vi "SPD Single Point Test Launcher.vi"() -> ()   [LabVIEW 2018]
uses:
  SPD Stand/typedefs/SPD.Stand state.ctl
  SPD Stand/typedefs/SPD.Stand Tabs.ctl
  Instruments/SPD HID Interface/hidSPDLibForLabView/LibVIs/hidSPD Controls/hidSPD SPD Type.ctl
  Instruments/SPD HID Interface/hidSPDLibForLabView/hidSPDLibForLabView.lvlib
  SPD Stand/typedefs/SPD.Queues.ctl
  SPD Stand/typedefs/SPD.Meas Grid.ctl
  <vilib>/Utility/config.llb/Config Data RefNum.ctl
  <vilib>/Utility/config.llb/NI_LVConfig.lvlib
  SPD Stand/ConfigFile/SPD.Config File ctrl.ctl
  SPD Stand/typedefs/SPD.Events.ctl
  Instruments/LeCroy SDA830/typedefs/LeCroy.Session.ctl
  Instruments/KeySight 8164B/KeySight 8164B LAN InstrLib/typedefs/KeySight 8164B control.ctl
  Instruments/KeySight 8164B/KeySight 8164B LAN InstrLib.lvlib
  Instruments/KeySight 53230A/typedefs/FreqC.Session.ctl
  Instruments/KC705 DevBoard/typedefs/DevB.Session.ctl
  Instruments/SPD HID Interface/hidSPDLibForLabView/LibVIs/hidSPD Controls/hidSPD Controller.ctl
  Instruments/SPD HID Interface/hidSPDLibForLabView/LibVIs/hidSPD Controls/hidSPD Device Session.ctl
  SPD Stand/typedefs/SPD.Stand Ctrl.ctl
  Instruments/SPD HID Interface/hidSPDLibForLabView/LibVIs/hidSPD Controls/hidSPD.STB Frequency.ctl
  Instruments/SPD HID Interface/hidSPDLibForLabView/LibVIs/hidSPD Controls/hidSPD SPD Diod Case.ctl
  Instruments/SPD HID Interface/hidSPDLibForLabView/LibVIs/hidSPD Controls/hidSPD.SPD specification.ctl
panel:
  out "Console":string caption="Консоль"
  out "test tabs":T1
  in  "HW.Ignore Equipment Tests":bool
  out "HW.KC Selftest":bool caption="Пройдено"
  in  "HW.KC705 Test":bool
  out "HW.PowerSource Selftest":bool caption="Пройдено"
  in  "HW.PowerSource Test":bool
  out "HW.Laser Selftest":bool caption="Пройдено"
  in  "HW.Laser Test":bool
  out "HW.Scope Selftest":bool caption="Пройдено"
  in  "HW.Scope Test":bool
  out "HW.8164B Selftest":bool caption="Пройдено"
  in  "HW.8164B Test":bool
  out "HW.FreqC Selftest":bool caption="Пройдено"
  in  "HW.FreqC Test":bool
  in  "Equipment.Connect":bool
  out "DevBSession.connected":bool caption="КС705"
  out "8164BSession.connected":bool caption="8164B"
  out "FreqCSession.connected":bool caption="Частотомер"
  out "LeCroySession.connected":bool caption="Осциллограф"
  in  "SPD.Type":T2=enum."Free Run" caption="Тип детектора"
  out "Diod T":sgl(graph) caption="Температура Диода"
  out "Heatsinck T":sgl(graph) caption="Температура Радиатора"
  in  "SPD.connect":bool
  out "hidSPDSession.connected":bool caption="Детектор подключен"
  out "spdDeviceSession.spdName":string caption="Имя Детектора"
  out "SPD.ready":bool caption="Вышел на режим"
  in  "TSet":sgl=-45.0 format="%#_g, Град С"
  in  "HV_bias":sgl=40.0 format="%#_g, В"
  in  "SPD.write":bool caption="Записать"
  out "PhaseTestProgress":dbl(slide) scale=0.0..1.0
  out "PhaseSetupGraph":cluster{dbl[], dbl[]}(graph) caption="Настройка Фазы Строба"
  out "HV_biasSetupGraph":cluster{dbl[], dbl[]}(graph) caption="Настройка Напряжения Смещения"
  out "Test.01_NoPulses Pass":bool caption="Отсутствие импульсов"
  in  "SPD.Tests":bool
  out "HV_BiasTestProgress":dbl(slide) scale=0.0..1.0
  out "Current Meas Progress":dbl(slide) caption="Измерение QE и TR" scale=0.0..1.0
  in  "Meas":bool
  out "Overall Meas Progress":dbl(slide) caption="Температура 1 из 1" scale=0.0..1.0
  out "Meas Time, min":dbl=nan format="%.2f"
  in  "SPMeas.Temprature":dbl=-45.0 caption="Температура"
  in  "SPMeas.Strobe_code":dbl=900.0 caption="Амплитуда Строба"
  in  "SPMeas.HV_bias":dbl=76.9 caption="Напряжение Смещения"
  out "Error Out":errorcluster
  out "SPD.Result":T3
  out "HW.Error Out":errorcluster
  in  "App.stop":bool
  in  "Back":bool
  in  "Next":bool
  # "Расширенные тесты оборудования"
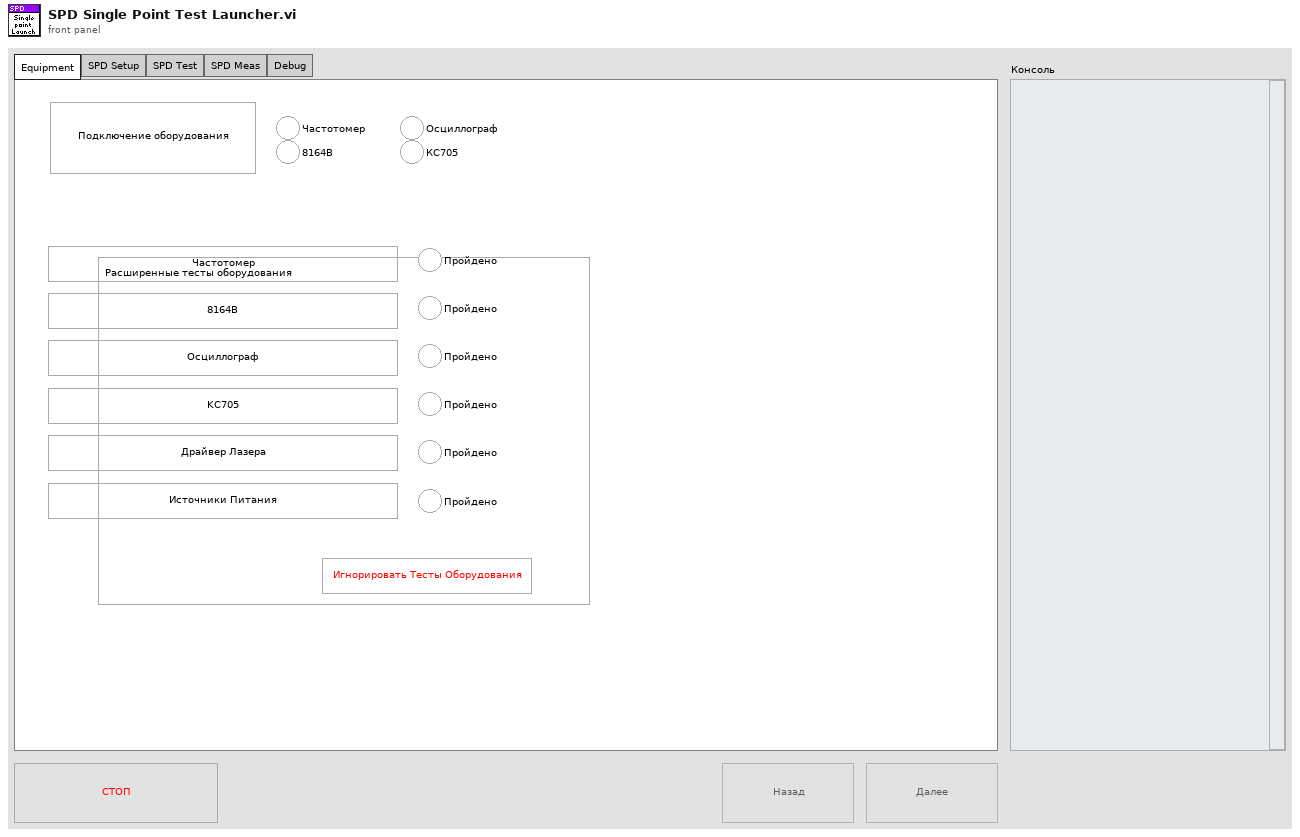
[diagram p1: front panel]
types:
  T1 = typedef "SPD.Stand Tabs.ctl" = enum32{"Equipment", "SPD Setup", "SPD Test", "SPD Meas", "Debug"}
  T2 = typedef "hidSPDLibForLabView.lvlib/hidSPD SPD Type.ctl" = enum16{"Unknown", "Free Run", "Gate"}
  T3 = typedef "SPD.Meas Grid.ctl" = cluster{"DateTime":string, "DT":dbl[], "Insensitivity":dbl[], "Temprature":dbl[], "Stb_code":dbl[], "HV_Bias":dbl[][][][]}
  T4 = typedef "SPD.Stand Ctrl.ctl" = cluster{"spdDeviceSession":T5, "DevBSession":T10, "FreqCSession":T11, "8164BSession":T12, "LeCroySession":T13, "Events":T14, "configFile":T15, "SPD.Meas Grid":T3, "SPD.Queues":T17, "Console":refnum<vi>}
  T5 = typedef "hidSPDLibForLabView.lvlib/hidSPD Device Session.ctl" = cluster{"spdRef":u64, "connected":bool, "spdName":string, "specification":T6, "hidSPD.Controller":T9, "hidSPD.Sturtup Values":T9}
  T6 = typedef "hidSPDLibForLabView.lvlib/hidSPD.SPD specification.ctl" = cluster{"diod case":T7, "type":T2, "frequency":T8}
  T7 = typedef "hidSPDLibForLabView.lvlib/hidSPD SPD Diod Case.ctl" = enum16{"Unknown", "default", "butterfly"}
  T8 = typedef "hidSPDLibForLabView.lvlib/hidSPD.STB Frequency.ctl" = enum16{"Unknown", "312", "1250"}
  T9 = typedef "hidSPDLibForLabView.lvlib/hidSPD Controller.ctl" = cluster{"TSet":sgl, "HV_bias":sgl, "DDS_stb_code":u16}
  T10 = typedef "DevB.Session.ctl" = cluster{"DevBRef":refnum<visa-resource-name>, "connected":bool}
  T11 = typedef "FreqC.Session.ctl" = cluster{"FreqCRef":refnum<visa-resource-name>, "timeout":dbl, "Gate":dbl, "connected":bool}
  T12 = typedef "KeySight 8164B LAN InstrLib.lvlib/KeySight 8164B control.ctl" = cluster{"Connection ID":refnum<k5>, "Connected":bool, "Info":string, "Slots Info":string[]}
  T13 = typedef "LeCroy.Session.ctl" = cluster{"LeCroySession":refnum<visa-resource-name>, "connected":bool}
  T14 = typedef "SPD.Events.ctl" = cluster{"DCRTest":refnum<user-event>, "Stop":refnum<user-event>}
  T15 = typedef "SPD.Config File ctrl.ctl" = cluster{"configFile ref":T16, "configFile path":path, "equipmentFile ref":T16}
  T16 = typedef "NI_LVConfig.lvlib/Config Data RefNum.ctl" = refnum<k1>
  T17 = typedef "SPD.Queues.ctl" = cluster{"state queue":refnum<queue>}
  T18 = enum8{"Enabled", "Disabled", "Disabled and Grayed Out"}
  T19 = typedef "SPD.Stand state.ctl" = enum16{"idle", "HW.Conect", "HW.FreqC selftest", "HW.8164B selftest", "HW.Scope selftest", "HW.KC705 selftest", "HW.Laser test", "HW.Power source test", "SPD.connect", "SPD.set type", "SPD.write", "SPD.read", "SPD.tests", "Btf.DT&Insens", "Meas.Grid update", "Meas", "App.Handle Error", "App.Stop"}
  T20 = typedef "hidSPDLibForLabView.lvlib/hidSPD SPD Type.ctl" = enum16{"Unknown", "Free Run", "Gate_312", "Gate_1250"}
  T21 = typedef "SPD.Meas Result.ctl" = cluster{"HV_Bias":dbl[][][], "Stb_code":dbl[], "Temprature":dbl[], "Data":dbl[][][][], "DateTime":string}
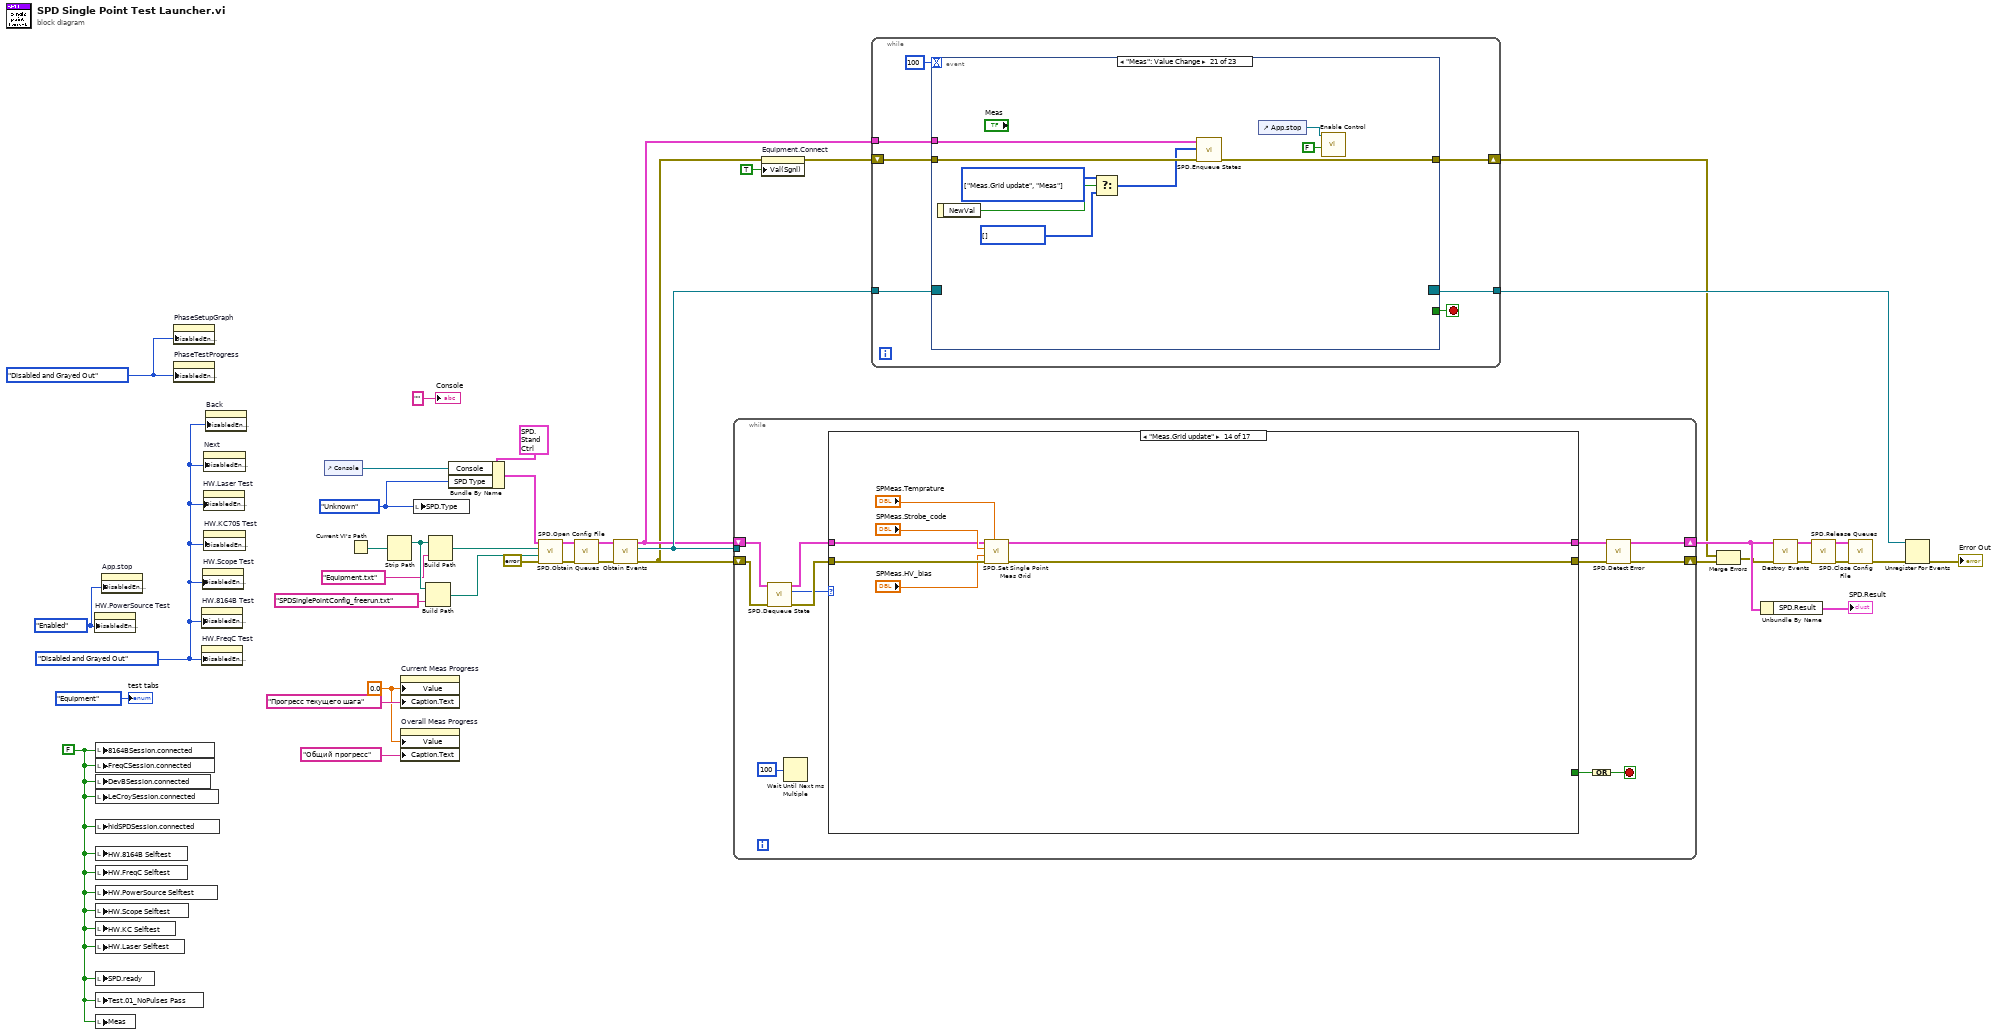
[diagram p0: block diagram]
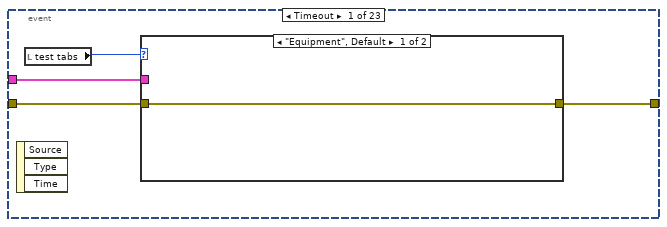
[diagram p2: hidden frame]
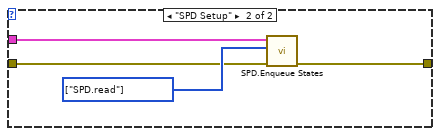
[diagram p3: hidden frame]
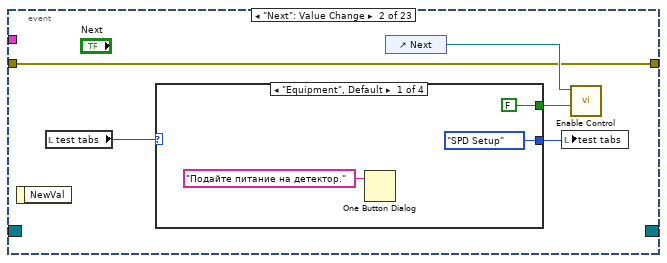
[diagram p4: hidden frame]
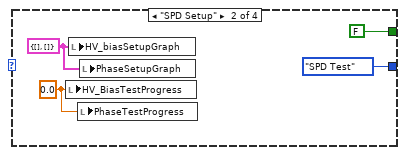
[diagram p5: hidden frame]
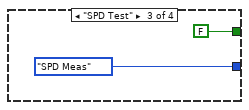
[diagram p6: hidden frame]
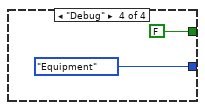
[diagram p7: hidden frame]
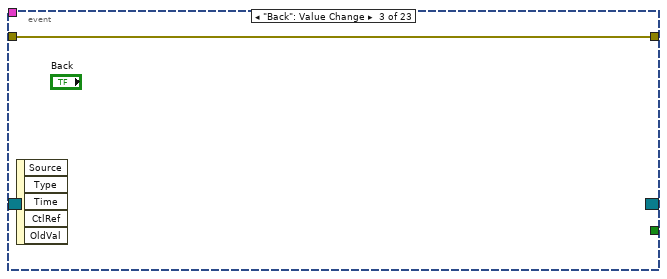
[diagram p8: hidden frame]
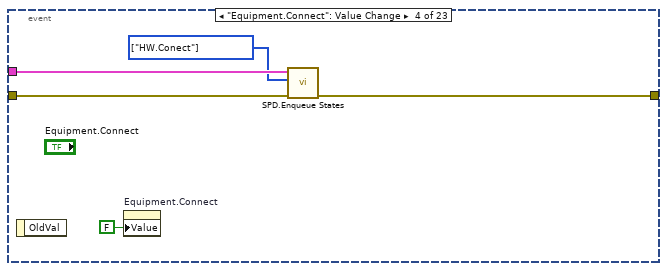
[diagram p9: hidden frame]
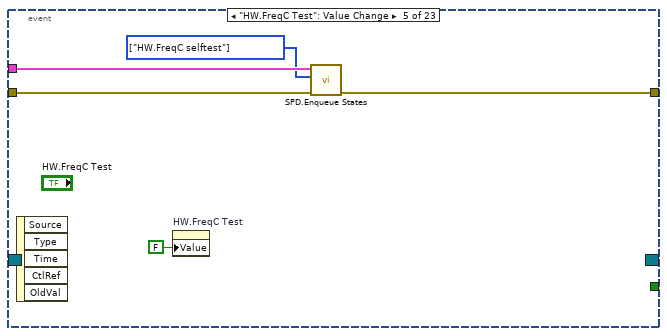
[diagram p10: hidden frame]
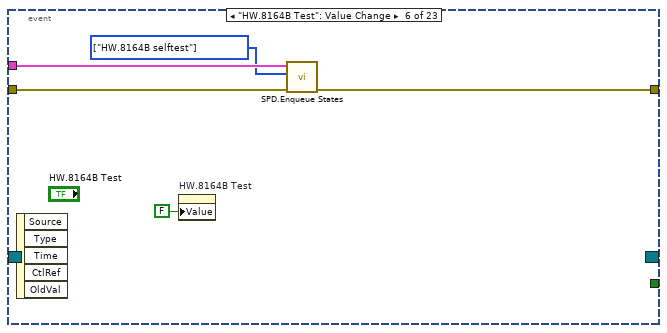
[diagram p11: hidden frame]
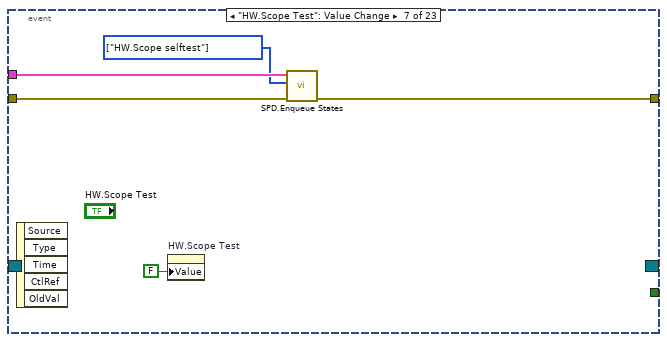
[diagram p12: hidden frame]
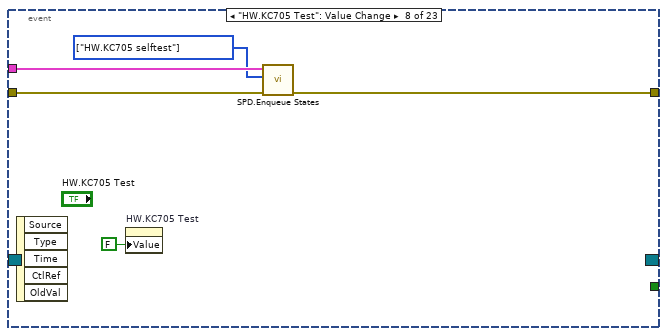
[diagram p13: hidden frame]
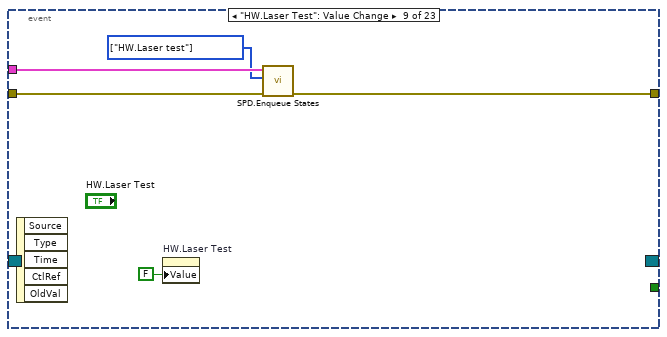
[diagram p14: hidden frame]
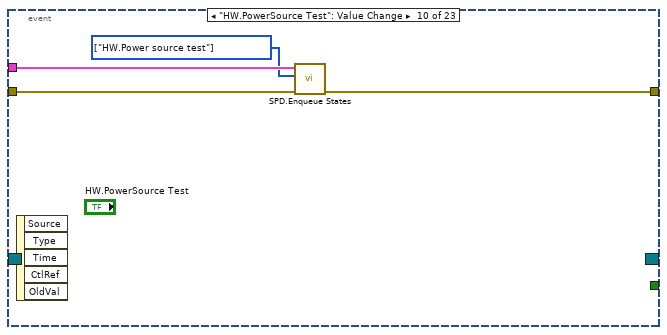
[diagram p15: hidden frame]
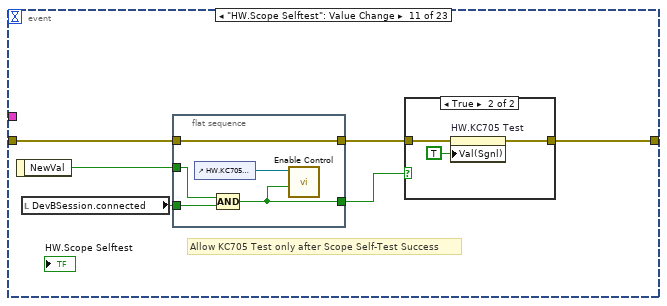
[diagram p16: hidden frame]
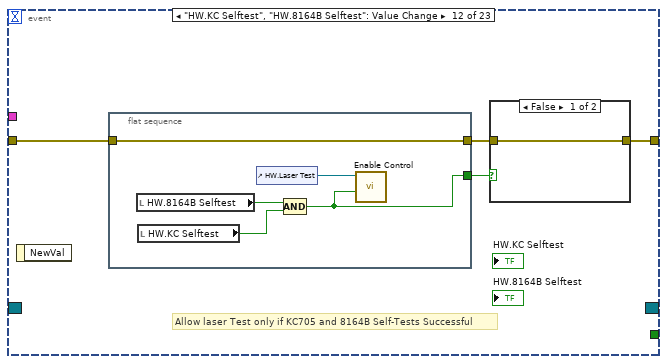
[diagram p18: hidden frame]
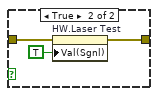
[diagram p19: hidden frame]
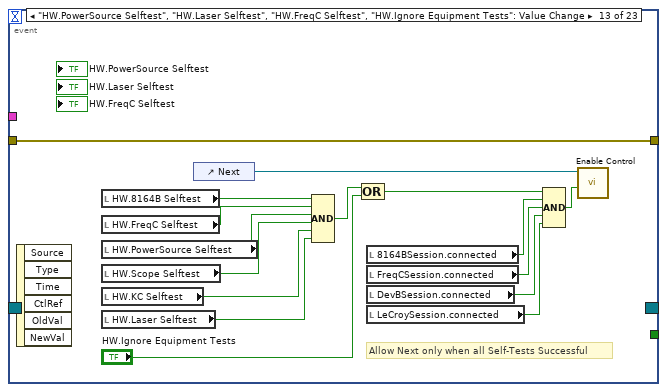
[diagram p20: hidden frame]
diagram:
  w2 = 0.0 ("Current Meas Progress")
  w4 = hidSPD_SPD_Type."Unknown" ("spdDeviceSession.SPD Type")
  w10 = T18."Disabled and Grayed Out" ("Disabled")
  w5 = T18."Enabled" ("Disabled")
  w33 = FALSE ("8164BSession.connected")
  w38 = T18."Disabled and Grayed Out" ("Disabled")
  n1 = property on="HW.PowerSource Test" class="Bool"("DisabledEnum"=w5) -> ()  [unwired: 2 in, 2 out]
  n2 = local write "8164BSession.connected"(w33) -> ()
  n3 = local write "FreqCSession.connected"(w33) -> ()
  n4 = local write "DevBSession.connected"(w33) -> ()
  n5 = local write "LeCroySession.connected"(w33) -> ()
  n6 = local write "hidSPDSession.connected"(w33) -> ()
  n7 = local write "HW.8164B Selftest"(w33) -> ()
  n8 = local write "HW.FreqC Selftest"(w33) -> ()
  n9 = local write "HW.PowerSource Selftest"(w33) -> ()
  n10 = local write "HW.Scope Selftest"(w33) -> ()
  n11 = local write "HW.KC Selftest"(w33) -> ()
  n12 = local write "HW.Laser Selftest"(w33) -> ()
  n13 = local write "SPD.ready"(w33) -> ()
  n14 = local write "Test.01_NoPulses Pass"(w33) -> ()
  n15 = local write "Meas"(w33) -> ()
  n16 = property on="App.stop" class="Bool"("DisabledEnum"=w5) -> ()  [unwired: 2 in, 2 out]
  n17 = property on="PhaseSetupGraph" class="XYGraph (strict)"("DisabledEnum"=w10) -> ()  [unwired: 2 in, 2 out]
  n18 = property on="PhaseTestProgress" class="Slide (strict)"("DisabledEnum"=w10) -> ()  [unwired: 2 in, 2 out]
  n19 = property on="HW.8164B Test" class="Bool (strict)"("DisabledEnum"=w38) -> ()  [unwired: 2 in, 2 out]
  n20 = property on="HW.FreqC Test" class="Bool (strict)"("DisabledEnum"=w38) -> ()  [unwired: 2 in, 2 out]
  n21 = property on="HW.Scope Test" class="Bool (strict)"("DisabledEnum"=w38) -> ()  [unwired: 2 in, 2 out]
  n22 = property on="HW.Laser Test" class="Bool (strict)"("DisabledEnum"=w38) -> ()  [unwired: 2 in, 2 out]
  n23 = property on="Next" class="Bool"("DisabledEnum"=w38) -> ()  [unwired: 2 in, 2 out]
  n24 = property on="HW.KC705 Test" class="Bool (strict)"("DisabledEnum"=w38) -> ()  [unwired: 2 in, 2 out]
  n25 = property on="Back" class="Bool"("DisabledEnum"=w38) -> ()  [unwired: 2 in, 2 out]
  n26 = control-ref of="Console"() -> (w13:refnum<vi>)
  n27 = Current VI's Path() -> (path=w37:path)
  n28 = Strip Path(path=w37) -> (stripped path=w9:path)  [unwired: 1 out]
  n29 = property on="Current Meas Progress" class="Slide (strict)"("Value"=w2, "Caption.Text"="Прогресс текущего шага") -> ()  [unwired: 2 in, 2 out]
  n30 = property on="Overall Meas Progress" class="Slide (strict)"("Value"=w2, "Caption.Text"="Общий прогресс") -> ()  [unwired: 2 in, 2 out]
  n31 = local write "SPD.Type"(w4) -> ()
  n32 = Build Path(base path=w9, name or relative path="SPDSinglePointConfig_freerun.txt") -> (appended path=w6:path)
  n33 = Build Path(base path=w9, name or relative path="Equipment.txt") -> (appended path=w7:path)
  n34 = Bundle By Name(cluster=T4 {"spdDeviceSession"={"spdRef"=0, "connected"=FALSE, "spdName"="", "specification"={"diod case"=enum."default", "type"=enum."Unknown", "frequency"=enum."Unknown"}, "hidSPD.Controller"={"TSet"=0.0, "HV_bias"=0.0, "DDS_stb_code"=0}, "hidSPD.Sturtup Values"={"TSet"=0.0, "HV_bias"=0.0, "DDS_stb_code"=0}}, "DevBSession"={"DevBRef"="", "connected"=FALSE}, "FreqCSession"={"FreqCRef"="", "timeout"=0.0, "Gate"=0.0, "connected"=FALSE}, "8164BSession"={"Connection ID"=refnum, "Connected"=FALSE, "Info"="", "Slots Info"=[]}, "LeCroySession"={"LeCroySession"="", "connected"=FALSE}, "Events"={"DCRTest"=refnum, "Stop"=refnum}, "configFile"={"configFile ref"=refnum, "configFile path"=path "", "equipmentFile ref"=refnum}, "SPD.Meas Grid"={"DateTime"="", "DT"=[], "Insensitivity"=[], "Temprature"=[], "Stb_code"=[], "HV_Bias"=[]}, "SPD.Queues"={"state queue"=refnum}, "Console"=refnum} ("SPD.Stand Ctrl in"), "Console"=w13, "SPD Type"=w4) -> (w14:T4)
  n35 = call "SPD.Open Config File.vi"("Error In"=errorcluster {"status"=FALSE, "code"=0, "source"=""}, "config file path"=w6, "equipment file path"=w7, "SPD.Stand Ctrl in"=w14) -> ("Error Out"=w29:errorcluster, "SPD.Stand Ctrl out"=w30:T4)  [unwired: 6 in]
  n36 = call "SPD.Obtain Queues.vi"("Error In"=w29, "SPD.Stand Ctrl in"=w30) -> ("Error Out"=w28:errorcluster, "SPD.Stand Ctrl out"=w23:T4)  [unwired: 8 in]
  n37 = call "Obtain Events.vi"("Error In"=w28, "SPD.Stand Ctrl in"=w23) -> ("Error Out"=w12:errorcluster, "Event Registration Refnum"=w22:refnum<event-registration>, "SPD.Stand Ctrl out"=w20:T4)  [unwired: 7 in]
  n38 = while {
    shift-right: [w43] -> w32
    shift-left: w20 -> [w51]
    shift-right: [w42] -> w39
    shift-left: w12 -> [w50]
    tunnel: w22 -> [_]
    stop <- w52 stop-if-true
    n39 = call "SPD.Dequeue State.vi"("Error In"=w50, "SPD.Stand Ctrl in"=w51) -> ("Error Out"=w48:errorcluster, "SPD.state"=w47:T19, "SPD.Stand Ctrl out"=w49:T4)  [unwired: 7 in]
    n40 = Wait Until Next ms Multiple(millisecond multiple=u32 100) -> ()  [unwired: 1 out]
    n41 = case shown="\"Meas.Grid update\"" w47 {
      tunnel: [_ _ _ _ _ _ _ _ _ _ _ _ _ _ _ _ TRUE] -> w53
      tunnel: [w55 w60 w77 w84 w89 w93 w97 w103 w110 w120 w132 w138 w155 w166 w175 w196 w199] -> w45
      tunnel: [w54 w56 w74 w80 w87 w92 w98 w102 w111 w122 w131 w137 w158 w167 w179 errorcluster {"status"=FALSE, "code"=0, "source"=""} ("Error Out") w200] -> w44
      tunnel: w49 -> [w55 w62 w78 w85 w90 w95 w100 w105 w113 w128 w134 w143 w157 w165 w177 w198 w203]
      tunnel: w48 -> [w54 w61 w76 w83 w88 w94 w99 w104 w112 w119 w133 w142 w156 w164 w176 w197 w202]
      frame "idle", Default {
      }
      frame "HW.Conect" {
        n42 = call "SPD.Connection Test.vi"("Error In"=w61, "SPD.Stand Ctrl in"=w62) -> ("Error Out"=w58:errorcluster, "SPD.Stand Ctrl out"=w60:T4)  [unwired: 7 in, 1 out]
        n43 = flat-sequence {
          tunnel: w60 -> [w64]
          tunnel: w58 -> [w63]
          tunnel: [w63] -> w57
          frame #0 {
            n44 = control-ref of="HW.FreqC Test"() -> (w71:refnum<vi>)
            n45 = control-ref of="HW.8164B Test"() -> (w69:refnum<vi>)
            n46 = control-ref of="HW.Scope Test"() -> (w68:refnum<vi>)
            n47 = Unbundle By Name(w64) -> ("DevBSession.connected"=→"DevBSession.connected":bool, "FreqCSession.connected"=w70:bool, "8164BSession.Connected"=w65:bool, "LeCroySession.connected"=w67:bool)
            "FreqCSession.connected" <- w70
            "8164BSession.connected" <- w65
            "LeCroySession.connected" <- w67
            n48 = call "Enable Control.vi"("enable"=w70, "Control"=w71) -> ()  [unwired: 10 in]
            n49 = call "Enable Control.vi"("enable"=w65, "Control"=w69) -> ()  [unwired: 10 in]
            n50 = call "Enable Control.vi"("enable"=w67, "Control"=w68) -> ()  [unwired: 10 in]
          }
        }
        n51 = property on="HW.FreqC Test" class="Bool (strict)"(error in=w57, "Val(Sgnl)"=TRUE ("Value (Signaling)")) -> (error out=w56:errorcluster)  [unwired: 1 in, 1 out]
      }
      frame "HW.FreqC selftest" {
        n52 = call "SPD.FreqC Self-Test.vi"("Error In"=w76, "SPD.Stand Ctrl in"=w78) -> ("Error Out"=w73:errorcluster, "ok"=w79:bool, "SPD.Stand Ctrl out"=w77:T4)  [unwired: 7 in]
        n53 = property on="HW.FreqC Selftest" class="Bool (strict)"(error in=w73, "Val(Sgnl)"=w79) -> (error out=w72:errorcluster)  [unwired: 1 in, 1 out]
        n54 = property on="HW.8164B Test" class="Bool (strict)"(error in=w72, "Val(Sgnl)"=TRUE ("Value (Signaling)")) -> (error out=w74:errorcluster)  [unwired: 1 in, 1 out]
      }
      frame "HW.8164B selftest" {
        n55 = call "SPD.8164B Self-Test.vi"("Error In"=w83, "SPD.Stand Ctrl in"=w85) -> ("Error Out"=w81:errorcluster, "ok"=w86:bool, "SPD.Stand Ctrl out"=w84:T4)  [unwired: 7 in]
        n56 = property on="HW.8164B Selftest" class="Bool (strict)"("Val(Sgnl)"=w86) -> ()  [unwired: 2 in, 2 out]
        n57 = property on="HW.Scope Test" class="Bool (strict)"(error in=w81, "Val(Sgnl)"=TRUE ("Value (Signaling)")) -> (error out=w80:errorcluster)  [unwired: 1 in, 1 out]
      }
      frame "HW.Scope selftest" {
        n58 = call "SPD.LeCroy Self-Test.vi"("Error In"=w88, "SPD.Stand Ctrl in"=w90) -> ("Error Out"=w87:errorcluster, "ok"=w91:bool, "SPD.Stand Ctrl out"=w89:T4)  [unwired: 7 in]
        n59 = property on="HW.Scope Selftest" class="Bool (strict)"("Val(Sgnl)"=w91) -> ()  [unwired: 2 in, 2 out]
      }
      frame "HW.KC705 selftest" {
        n60 = call "SPD.KC705 Test.vi"("Error In"=w94, "SPD.Stand Ctrl in"=w95) -> ("Error Out"=w92:errorcluster, "ok"=w96:bool, "SPD.Stand Ctrl out"=w93:T4)  [unwired: 7 in]
        n61 = property on="HW.KC Selftest" class="Bool (strict)"("Val(Sgnl)"=w96) -> ()  [unwired: 2 in, 2 out]
      }
      frame "HW.Laser test" {
        n62 = call "SPD.Liser Driver Test.vi"("Error In"=w99, "SPD.Stand Ctrl in"=w100) -> ("Error Out"=w98:errorcluster, "ok"=w101:bool, "SPD.Stand Ctrl out"=w97:T4)  [unwired: 7 in]
        n63 = property on="HW.Laser Selftest" class="Bool (strict)"("Val(Sgnl)"=w101) -> ()  [unwired: 2 in, 2 out]
      }
      frame "HW.Power source test" {
        n64 = call "SPD.PowerSource Test.vi"("Error In"=w104, "SPD.Stand Ctrl in"=w105) -> ("Error Out"=w102:errorcluster, "ok"=w106:bool, "SPD.Stand Ctrl out"=w103:T4)  [unwired: 7 in]
        n65 = property on="HW.PowerSource Selftest" class="Bool (strict)"("Val(Sgnl)"=w106) -> ()  [unwired: 2 in, 2 out]
      }
      frame "SPD.connect" {
        n66 = call "SPD.Detector Connection Test.vi"("Error In"=w112, "SPD.Stand Ctrl in"=w113) -> ("Error Out"=w111:errorcluster, "SPD.Stand Ctrl out"=w110:T4)  [unwired: 7 in, 1 out]
        n67 = Unbundle By Name(w110) -> ("spdDeviceSession.connected"=→"hidSPDSession.connected":bool, "spdDeviceSession.spdName"=→"spdDeviceSession.spdName":string, "spdDeviceSession.hidSPD.Controller.TSet"=w109:sgl, "spdDeviceSession.hidSPD.Controller.HV_bias"=w108:sgl, "SPD Type"=w107:T20)
        n68 = local write "TSet"(w109) -> ()
        n69 = local write "HV_bias"(w108) -> ()
        n70 = local write "SPD.Type"(w107) -> ()
      }
      frame "SPD.set type" {
        n71 = control-ref of="PhaseTestProgress"() -> (w126:refnum<vi>)
        n72 = control-ref of="PhaseSetupGraph"() -> (w124:refnum<vi>)
        n73 = case shown="\"Gate\"" "SPD.Type" {
          tunnel: [T18."Disabled and Grayed Out" ("Disabled") T18."Enabled" ("Disabled")] -> w123
          frame "Free Run", Default {
          }
          frame "Gate" {
          }
        }
        n74 = Bundle By Name(cluster=w128, "SPD Type"="SPD.Type") -> (w121:T4)
        n75 = call "SPD.Update Config File.vi"(6:"SPDSinglePointConfig_freerun.txt" ("freerun SPD config"), "Error In"=w119, 10:"SPDSinglePointConfig_strobe_312.txt" ("gated SPD config"), "SPD.Stand Ctrl in"=w121) -> ("Error Out"=w118:errorcluster, "SPD.Stand Ctrl out"=w120:T4)  [unwired: 6 in]
        n76 = property on="Property Node" class="Slide (strict)"(reference=w126, error in=w118, "DisabledEnum"=w123) -> (error out=w125:errorcluster)  [unwired: 1 out]
        n77 = property on="Property Node" class="XYGraph (strict)"(reference=w124, error in=w125, "DisabledEnum"=w123) -> (error out=w122:errorcluster)  [unwired: 1 out]
      }
      frame "SPD.write" {
        n78 = call "SPD.Write SPD Controller Setup.vi"("Error In"=w133, "HV_bias"="HV_bias", "TSet"="TSet", "SPD.Stand Ctrl in"=w134) -> ("Error Out"=w131:errorcluster, "SPD.Stand Ctrl out"=w132:T4)  [unwired: 6 in]
      }
      frame "SPD.read" {
        n79 = call "SPD.Read SPD Telemetry.vi"("Error In"=w142, "SPD.Stand Ctrl in"=w143) -> ("Error Out"=w137:errorcluster, "Diod Temprature"=→"Diod T":sgl, "Heatsink Temprature"=→"Heatsinck T":sgl, "SPD.Stand Ctrl out"=w138:T4, "Ready"=w139:bool)  [unwired: 5 in]
        n80 = property on="SPD.ready" class="Bool (strict)"("Val(Sgnl)"=w139) -> ()  [unwired: 2 in, 2 out]
      }
      frame "SPD.tests" {
        n81 = control-ref of="PhaseTestProgress"() -> (w145:refnum<vi>)
        n82 = control-ref of="PhaseSetupGraph"() -> (w144:refnum<vi>)
        n83 = control-ref of="HV_biasSetupGraph"() -> (w149:refnum<vi>)
        n84 = control-ref of="HV_BiasTestProgress"() -> (w148:refnum<vi>)
        n85 = call "SPD.Tests.vi"("Phase Graph"=w144, "HV_Bias Graph"=w149, "Phase Progress"=w145, "HV_Bias Progress"=w148, "Error In"=w156, "SPD.Stand Ctrl in"=w157) -> ("Error Out"=w151:errorcluster, "pass"=w152:bool, "SPD.Stand Ctrl out"=w155:T4)  [unwired: 3 in]
        n86 = property on="Test.01_NoPulses Pass" class="Bool (strict)"(error in=w151, "Val(Sgnl)"=w152) -> (error out=w150:errorcluster)  [unwired: 1 in, 1 out]
        n87 = control-ref of="App.stop"() -> (w159:refnum<vi>)
        n88 = flat-sequence {
          tunnel: [w160] -> w158
          tunnel: w159 -> [w162]
          tunnel: w150 -> [w160]
          frame #0 {
            n89 = call "Enable Control.vi"("enable"=TRUE, "Control"=w162) -> ()  [unwired: 10 in]
          }
        }
        "HV_biasSetupGraph" <- cluster{dbl[], dbl[]} {[], []} ("HV_biasSetupGraph")
        "HV_BiasTestProgress" <- 0.0 ("HV_BiasTestProgress")
        "PhaseSetupGraph" <- cluster{dbl[], dbl[]} {[], []} ("PhaseSetupGraph")
        "PhaseTestProgress" <- 0.0 ("PhaseTestProgress")
      }
      frame "Meas.Grid update" {
        n90 = call "SPD.Set Single Point Meas Grid.vi"("Temprature"="SPMeas.Temprature", "Error In"=w164, "HV_bias"="SPMeas.HV_bias", "Strobe_code"="SPMeas.Strobe_code", "SPD.Stand Ctrl in"=w165) -> ("Error Out"=w167:errorcluster, "SPD.Stand Ctrl out"=w166:T4)  [unwired: 5 in]
      }
      frame "Meas" {
        w188 = 0.0 ("MeasProgress")
        n91 = control-ref of="Meas"() -> (w173:refnum<vi>)
        n92 = control-ref of="Current Meas Progress"() -> (w172:refnum<vi>)
        n93 = control-ref of="Overall Meas Progress"() -> (w171:refnum<vi>)
        n94 = flat-sequence {
          tunnel: [w193] -> w183
          tunnel: w176 -> [_]
          frame #0 {
            n95 = Tick Count (ms)() -> (millisecond timer value=w193:u32)
          }
        }
        n96 = property on="Meas Time, min" class="DigNum (strict)"("Value"=nan ("Grid Time")) -> ()  [unwired: 2 in, 2 out]
        n97 = call "SPD.Measurments Single Point.vi"("Current Progress"=w172, "Overall Progress"=w171, "Continue"=w173, "Error In"=w176, "SPD.Stand Ctrl in"=w177) -> ("Error Out"=w174:errorcluster, "pass"=w170:bool, "SPD.Stand Ctrl out"=w175:T4)  [unwired: 4 in]
        n98 = flat-sequence {
          tunnel: [w192] -> w186
          tunnel: w174 -> [_]
          frame #0 {
            n99 = Tick Count (ms)() -> (millisecond timer value=w192:u32)
          }
        }
        n100 = control-ref of="Next"() -> (w178:refnum<vi>)
        n101 = control-ref of="App.stop"() -> (w180:refnum<vi>)
        n102 = call "Enable Control.vi"("enable"=w170, "Control"=w178) -> ()  [unwired: 10 in]
        n103 = Subtract(x=w186, y=w183) -> (x-y=w185:u32)
        n104 = Compound Arithmetic op=MULTIPLY(w185, invert u32 1000 ("x"), invert 60.0 ("value")) -> (→"Meas Time, min":dbl)
        n105 = flat-sequence {
          tunnel: w174 -> [w191]
          tunnel: [w191] -> w179
          tunnel: w180 -> [w190]
          frame #0 {
            n106 = call "Enable Control.vi"("enable"=TRUE, "Control"=w190) -> ()  [unwired: 10 in]
          }
        }
        "Current Meas Progress" <- w188
        "Overall Meas Progress" <- w188
      }
      frame "App.Handle Error" {
        n107 = call "SPD.Error Handler.vi"("Error In"=w197, "SPD.Stand Ctrl in"=w198) -> ("Error Out"=→"HW.Error Out":errorcluster, "SPD.Stand Ctrl out"=w196:T4)  [unwired: 7 in, 1 out]
      }
      frame "App.Stop" {
        n108 = call "SPD.Disconnect HW.vi"("Error In"=w202, "SPD.Stand Ctrl in"=w203) -> ("Error Out"=w200:errorcluster, "SPD.Stand Ctrl out"=w199:T4)  [unwired: 7 in, 1 out]
      }
    }
    n109 = Compound Arithmetic op=OR(w53) -> (w52:bool)
    n110 = call "SPD.Detect Error.vi"("Error In"=w44, "SPD.Stand Ctrl in"=w45) -> ("Error Out"=w42:errorcluster, "SPD.Stand Ctrl out"=w43:T4)  [unwired: 8 in]
  }
  n111 = property on="Equipment.Connect" class="Bool (strict)"(error in=w12, "Val(Sgnl)"=TRUE) -> (error out=w16:errorcluster)  [unwired: 1 in, 1 out]
  n112 = while {
    tunnel: w20 -> [w207]
    tunnel: w22 -> [w210]
    tunnel: [w209] -> w21
    shift-right: [w205] -> w18
    shift-left: w16 -> [w206]
    stop <- w208 stop-if-true
    n113 = event shown="[20] \"Meas\": Value Change" {
      selector: w210 -> [_ _ _ _ _ _ _ _ _ _ _ _ _ _ _ _ _ _ _ _ _ _ _]
      dyn-events: [_ _ _ _ _ _ _ _ _ _ _ _ _ _ _ _ _ _ _ _ _ _ _] -> w209
      timeout: 100 -> [_ _ _ _ _ _ _ _ _ _ _ _ _ _ _ _ _ _ _ _ _ _ _]
      tunnel: [_ _ _ _ _ _ _ _ _ _ _ _ _ _ _ _ _ _ _ _ _ TRUE _] -> w208
      tunnel: w207 -> [w213 _ _ w241 w246 w251 w256 w261 w266 w270 _ _ _ w319 w323 w327 _ w336 _ w341 w351 w355 w359]
      tunnel: w206 -> [w212 w220 w236 w240 w245 w250 w255 w260 w265 w269 w274 w289 w314 w317 w321 w325 w330 w335 w338 w340 w350 w354 w360]
      tunnel: [w211 w220 w236 w237 w242 w247 w252 w257 w262 w267 w272 w287 w314 w315 w320 w324 w330 w331 w338 w339 w343 w352 w357] -> w205
      event Timeout {
        n114 = event-data() -> ()  [unwired: 1 in, 3 out]
        n115 = local read "test tabs"() -> (w214:T1)
        n116 = case shown="\"Equipment\", Default" w214 {
          tunnel: w213 -> [_ w218]
          tunnel: w212 -> [w215 w217]
          tunnel: [w215 w216] -> w211
          frame "Equipment", Default {
          }
          frame "SPD Setup" {
            w219 = T19[] [enum."SPD.read"] items=["idle", "HW.Conect", "HW.FreqC selftest", "HW.8164B selftest", "HW.Scope selftest", "HW.KC705 selftest", "HW.Laser test", "HW.Power source test", "SPD.connect", "SPD.set type", "SPD.write", "SPD.read", "SPD.tests", "Btf.DT&Insens", "Meas.Grid update", "Meas", "App.Handle Error", "App.Stop"] ("SPD.states")
            n117 = call "SPD.Enqueue States.vi"("Error In"=w217, "SPD.states"=w219, "SPD.Stand Ctrl in"=w218) -> ("Error Out"=w216:errorcluster)  [unwired: 7 in, 1 out]
          }
        }
      }
      event "Next": Value Change {
        n118 = event-data() -> ()  [unwired: 1 in, 1 out]
        n119 = local read "test tabs"() -> (w223:T1)
        n120 = case shown="\"Equipment\", Default" w223 {
          tunnel: [SPD.Stand_Tabs."SPD Setup" ("test tabs") SPD.Stand_Tabs."SPD Test" ("test tabs") SPD.Stand_Tabs."SPD Meas" ("test tabs") SPD.Stand_Tabs."Equipment" ("test tabs")] -> w224
          tunnel: [FALSE FALSE FALSE FALSE] -> w221
          frame "Equipment", Default {
            n121 = One Button Dialog(message="Подайте питание на детектор.") -> ()  [unwired: 1 in, 1 out]
          }
          frame "SPD Setup" {
            w228 = 0.0 ("HV_BiasTestProgress")
            w229 = cluster{dbl[], dbl[]} {[], []} ("HV_biasSetupGraph")
            n122 = local write "HV_BiasTestProgress"(w228) -> ()
            n123 = local write "HV_biasSetupGraph"(w229) -> ()
            n124 = local write "PhaseTestProgress"(w228) -> ()
            n125 = local write "PhaseSetupGraph"(w229) -> ()
          }
          frame "SPD Test" {
          }
          frame "Debug" {
          }
        }
        n126 = control-ref of="Next"() -> (w222:refnum<vi>)
        n127 = local write "test tabs"(w224) -> ()
        n128 = call "Enable Control.vi"("enable"=w221, "Control"=w222) -> ()  [unwired: 10 in]
      }
      event "Back": Value Change {
        n129 = event-data() -> ()  [unwired: 1 in, 5 out]
      }
      event "Equipment.Connect": Value Change {
        w239 = T19[] [enum."HW.Conect"] items=["idle", "HW.Conect", "HW.FreqC selftest", "HW.8164B selftest", "HW.Scope selftest", "HW.KC705 selftest", "HW.Laser test", "HW.Power source test", "SPD.connect", "SPD.set type", "SPD.write", "SPD.read", "SPD.tests", "Btf.DT&Insens", "Meas.Grid update", "Meas", "App.Handle Error", "App.Stop"] ("SPD.states")
        n130 = event-data() -> ()  [unwired: 1 in, 1 out]
        n131 = property on="Equipment.Connect" class="Bool (strict)"("Value"=FALSE ("Equipment.Connect")) -> ()  [unwired: 2 in, 2 out]
        n132 = call "SPD.Enqueue States.vi"("Error In"=w240, "SPD.states"=w239, "SPD.Stand Ctrl in"=w241) -> ("Error Out"=w237:errorcluster)  [unwired: 7 in, 1 out]
      }
      event "HW.FreqC Test": Value Change {
        w244 = T19[] [enum."HW.FreqC selftest"] items=["idle", "HW.Conect", "HW.FreqC selftest", "HW.8164B selftest", "HW.Scope selftest", "HW.KC705 selftest", "HW.Laser test", "HW.Power source test", "SPD.connect", "SPD.set type", "SPD.write", "SPD.read", "SPD.tests", "Btf.DT&Insens", "Meas.Grid update", "Meas", "App.Handle Error", "App.Stop"] ("SPD.states")
        n133 = event-data() -> ()  [unwired: 1 in, 5 out]
        n134 = property on="HW.FreqC Test" class="Bool (strict)"("Value"=FALSE ("HW.FreqC Test")) -> ()  [unwired: 2 in, 2 out]
        n135 = call "SPD.Enqueue States.vi"("Error In"=w245, "SPD.states"=w244, "SPD.Stand Ctrl in"=w246) -> ("Error Out"=w242:errorcluster)  [unwired: 7 in, 1 out]
      }
      event "HW.8164B Test": Value Change {
        w249 = T19[] [enum."HW.8164B selftest"] items=["idle", "HW.Conect", "HW.FreqC selftest", "HW.8164B selftest", "HW.Scope selftest", "HW.KC705 selftest", "HW.Laser test", "HW.Power source test", "SPD.connect", "SPD.set type", "SPD.write", "SPD.read", "SPD.tests", "Btf.DT&Insens", "Meas.Grid update", "Meas", "App.Handle Error", "App.Stop"] ("SPD.states")
        n136 = event-data() -> ()  [unwired: 1 in, 5 out]
        n137 = property on="HW.8164B Test" class="Bool (strict)"("Value"=FALSE ("HW.8164B Test")) -> ()  [unwired: 2 in, 2 out]
        n138 = call "SPD.Enqueue States.vi"("Error In"=w250, "SPD.states"=w249, "SPD.Stand Ctrl in"=w251) -> ("Error Out"=w247:errorcluster)  [unwired: 7 in, 1 out]
      }
      event "HW.Scope Test": Value Change {
        w254 = T19[] [enum."HW.Scope selftest"] items=["idle", "HW.Conect", "HW.FreqC selftest", "HW.8164B selftest", "HW.Scope selftest", "HW.KC705 selftest", "HW.Laser test", "HW.Power source test", "SPD.connect", "SPD.set type", "SPD.write", "SPD.read", "SPD.tests", "Btf.DT&Insens", "Meas.Grid update", "Meas", "App.Handle Error", "App.Stop"] ("SPD.states")
        n139 = event-data() -> ()  [unwired: 1 in, 5 out]
        n140 = property on="HW.Scope Test" class="Bool (strict)"("Value"=FALSE ("HW.Scope Test")) -> ()  [unwired: 2 in, 2 out]
        n141 = call "SPD.Enqueue States.vi"("Error In"=w255, "SPD.states"=w254, "SPD.Stand Ctrl in"=w256) -> ("Error Out"=w252:errorcluster)  [unwired: 7 in, 1 out]
      }
      event "HW.KC705 Test": Value Change {
        w259 = T19[] [enum."HW.KC705 selftest"] items=["idle", "HW.Conect", "HW.FreqC selftest", "HW.8164B selftest", "HW.Scope selftest", "HW.KC705 selftest", "HW.Laser test", "HW.Power source test", "SPD.connect", "SPD.set type", "SPD.write", "SPD.read", "SPD.tests", "Btf.DT&Insens", "Meas.Grid update", "Meas", "App.Handle Error", "App.Stop"] ("SPD.states")
        n142 = event-data() -> ()  [unwired: 1 in, 5 out]
        n143 = property on="HW.KC705 Test" class="Bool (strict)"("Value"=FALSE ("HW.KC705 Test")) -> ()  [unwired: 2 in, 2 out]
        n144 = call "SPD.Enqueue States.vi"("Error In"=w260, "SPD.states"=w259, "SPD.Stand Ctrl in"=w261) -> ("Error Out"=w257:errorcluster)  [unwired: 7 in, 1 out]
      }
      event "HW.Laser Test": Value Change {
        w264 = T19[] [enum."HW.Laser test"] items=["idle", "HW.Conect", "HW.FreqC selftest", "HW.8164B selftest", "HW.Scope selftest", "HW.KC705 selftest", "HW.Laser test", "HW.Power source test", "SPD.connect", "SPD.set type", "SPD.write", "SPD.read", "SPD.tests", "Btf.DT&Insens", "Meas.Grid update", "Meas", "App.Handle Error", "App.Stop"] ("SPD.states")
        n145 = event-data() -> ()  [unwired: 1 in, 5 out]
        n146 = property on="HW.Laser Test" class="Bool (strict)"("Value"=FALSE ("HW.Laser Test")) -> ()  [unwired: 2 in, 2 out]
        n147 = call "SPD.Enqueue States.vi"("Error In"=w265, "SPD.states"=w264, "SPD.Stand Ctrl in"=w266) -> ("Error Out"=w262:errorcluster)  [unwired: 7 in, 1 out]
      }
      event "HW.PowerSource Test": Value Change {
        w268 = T19[] [enum."HW.Power source test"] items=["idle", "HW.Conect", "HW.FreqC selftest", "HW.8164B selftest", "HW.Scope selftest", "HW.KC705 selftest", "HW.Laser test", "HW.Power source test", "SPD.connect", "SPD.set type", "SPD.write", "SPD.read", "SPD.tests", "Btf.DT&Insens", "Meas.Grid update", "Meas", "App.Handle Error", "App.Stop"] ("SPD.states")
        n148 = event-data() -> ()  [unwired: 1 in, 5 out]
        n149 = call "SPD.Enqueue States.vi"("Error In"=w269, "SPD.states"=w268, "SPD.Stand Ctrl in"=w270) -> ("Error Out"=w267:errorcluster)  [unwired: 7 in, 1 out]
      }
      event "HW.Scope Selftest": Value Change {
        # "Allow KC705 Test only after Scope Self-Test Success"
        n150 = event-data() -> ("NewVal"=w275:bool)  [unwired: 1 in]
        n151 = local read "DevBSession.connected"() -> (w276:bool)
        n152 = flat-sequence {
          tunnel: w276 -> [w285]
          tunnel: w275 -> [w283]
          tunnel: w274 -> [w282]
          tunnel: [w282] -> w273
          tunnel: [w281] -> w271
          frame #0 {
            n153 = control-ref of="HW.KC705 Test"() -> (w284:refnum<vi>)
            n154 = Compound Arithmetic op=AND(w283, w285) -> (w281:bool)
            n155 = call "Enable Control.vi"("enable"=w281, "Control"=w284) -> ()  [unwired: 10 in]
          }
        }
        n156 = case shown="True" w271 {
          tunnel: w273 -> [w277 w280]
          tunnel: [w277 w279] -> w272
          frame False {
          }
          frame True {
            n157 = property on="HW.KC705 Test" class="Bool (strict)"(error in=w280, "Val(Sgnl)"=TRUE ("Value (Signaling)")) -> (error out=w279:errorcluster)  [unwired: 1 in, 1 out]
          }
        }
      }
      event "HW.KC Selftest", "HW.8164B Selftest": Value Change {
        # "Allow laser Test only if KC705 and 8164B Self-Tests Successful"
        n158 = event-data() -> ()  [unwired: 1 in, 1 out]
        n159 = flat-sequence {
          tunnel: w289 -> [w295]
          tunnel: [w295] -> w288
          tunnel: [w294] -> w286
          frame #0 {
            n160 = local read "HW.8164B Selftest"() -> (w297:bool)
            n161 = local read "HW.KC Selftest"() -> (w298:bool)
            n162 = control-ref of="HW.Laser Test"() -> (w296:refnum<vi>)
            n163 = Compound Arithmetic op=AND(w297, w298) -> (w294:bool)
            n164 = call "Enable Control.vi"("enable"=w294, "Control"=w296) -> ()  [unwired: 10 in]
          }
        }
        n165 = case shown="False" w286 {
          tunnel: w288 -> [w290 w293]
          tunnel: [w290 w292] -> w287
          frame False {
          }
          frame True {
            n166 = property on="HW.Laser Test" class="Bool (strict)"(error in=w293, "Val(Sgnl)"=TRUE ("Value (Signaling)")) -> (error out=w292:errorcluster)  [unwired: 1 in, 1 out]
          }
        }
      }
      event "HW.PowerSource Selftest", "HW.Laser Selftest", "HW.FreqC Selftest", "HW.Ignore Equipment Tests": Value Change {
        # "Allow Next only when all Self-Tests Successful"
        n167 = event-data() -> ()  [unwired: 1 in, 6 out]
        n168 = local read "HW.8164B Selftest"() -> (w311:bool)
        n169 = local read "HW.FreqC Selftest"() -> (w310:bool)
        n170 = local read "HW.PowerSource Selftest"() -> (w309:bool)
        n171 = local read "HW.Scope Selftest"() -> (w308:bool)
        n172 = local read "HW.KC Selftest"() -> (w307:bool)
        n173 = local read "HW.Laser Selftest"() -> (w306:bool)
        n174 = control-ref of="Next"() -> (w312:refnum<vi>)
        n175 = Compound Arithmetic op=AND(w311, w310, w309, w308, w307, w306) -> (w313:bool)
        n176 = Compound Arithmetic op=OR(w313, "HW.Ignore Equipment Tests") -> (w304:bool)
        n177 = local read "8164BSession.connected"() -> (w303:bool)
        n178 = local read "FreqCSession.connected"() -> (w301:bool)
        n179 = local read "DevBSession.connected"() -> (w300:bool)
        n180 = local read "LeCroySession.connected"() -> (w299:bool)
        n181 = Compound Arithmetic op=AND(w304, w303, w301, w300, w299) -> (w302:bool)
        n182 = call "Enable Control.vi"("enable"=w302, "Control"=w312) -> ()  [unwired: 10 in]
      }
      event "SPD.connect": Value Change {
        w318 = T19[] [enum."SPD.connect"] items=["idle", "HW.Conect", "HW.FreqC selftest", "HW.8164B selftest", "HW.Scope selftest", "HW.KC705 selftest", "HW.Laser test", "HW.Power source test", "SPD.connect", "SPD.set type", "SPD.write", "SPD.read", "SPD.tests", "Btf.DT&Insens", "Meas.Grid update", "Meas", "App.Handle Error", "App.Stop"] ("SPD.states")
        n183 = event-data() -> ()  [unwired: 1 in, 6 out]
        n184 = property on="SPD.connect" class="Bool (strict)"("Value"=FALSE ("Equipment.Connect")) -> ()  [unwired: 2 in, 2 out]
        n185 = call "SPD.Enqueue States.vi"("Error In"=w317, "SPD.states"=w318, "SPD.Stand Ctrl in"=w319) -> ("Error Out"=w315:errorcluster)  [unwired: 7 in, 1 out]
      }
      event Value Change {
        w322 = T19[] [enum."SPD.set type"] items=["idle", "HW.Conect", "HW.FreqC selftest", "HW.8164B selftest", "HW.Scope selftest", "HW.KC705 selftest", "HW.Laser test", "HW.Power source test", "SPD.connect", "SPD.set type", "SPD.write", "SPD.read", "SPD.tests", "Btf.DT&Insens", "Meas.Grid update", "Meas", "App.Handle Error", "App.Stop"] ("SPD.states")
        n186 = event-data() -> ()  [unwired: 1 in, 6 out]
        n187 = call "SPD.Enqueue States.vi"("Error In"=w321, "SPD.states"=w322, "SPD.Stand Ctrl in"=w323) -> ("Error Out"=w320:errorcluster)  [unwired: 7 in, 1 out]
      }
      event "SPD.write": Value Change {
        w326 = T19[] [enum."SPD.write"] items=["idle", "HW.Conect", "HW.FreqC selftest", "HW.8164B selftest", "HW.Scope selftest", "HW.KC705 selftest", "HW.Laser test", "HW.Power source test", "SPD.connect", "SPD.set type", "SPD.write", "SPD.read", "SPD.tests", "Btf.DT&Insens", "Meas.Grid update", "Meas", "App.Handle Error", "App.Stop"] ("SPD.states")
        n188 = event-data() -> ()  [unwired: 1 in, 6 out]
        n189 = call "SPD.Enqueue States.vi"("Error In"=w325, "SPD.states"=w326, "SPD.Stand Ctrl in"=w327) -> ("Error Out"=w324:errorcluster)  [unwired: 7 in, 1 out]
      }
      event "SPD.ready": Value Change {
        n190 = event-data() -> ("NewVal"=w328:bool)  [unwired: 1 in]
        n191 = control-ref of="Next"() -> (w329:refnum<vi>)
        n192 = call "Enable Control.vi"("enable"=w328, "Control"=w329) -> ()  [unwired: 10 in]
      }
      event "SPD.Tests": Value Change {
        w337 = T19[] [enum."SPD.tests"] items=["idle", "HW.Conect", "HW.FreqC selftest", "HW.8164B selftest", "HW.Scope selftest", "HW.KC705 selftest", "HW.Laser test", "HW.Power source test", "SPD.connect", "SPD.set type", "SPD.write", "SPD.read", "SPD.tests", "Btf.DT&Insens", "Meas.Grid update", "Meas", "App.Handle Error", "App.Stop"] ("SPD.states")
        n193 = event-data() -> ()  [unwired: 1 in, 1 out]
        n194 = property on="SPD.Tests" class="Bool (strict)"("Value"=FALSE ("Test.01_NoPulses")) -> ()  [unwired: 2 in, 2 out]
        n195 = call "SPD.Enqueue States.vi"("Error In"=w335, "SPD.states"=w337, "SPD.Stand Ctrl in"=w336) -> ("Error Out"=w331:errorcluster)  [unwired: 7 in, 1 out]
        n196 = control-ref of="App.stop"() -> (w334:refnum<vi>)
        n197 = call "Enable Control.vi"("enable"=FALSE, "Control"=w334) -> ()  [unwired: 10 in]
      }
      event "Test.01_NoPulses Pass": Value Change {
        n198 = event-data() -> ()  [unwired: 1 in, 1 out]
      }
      event "SPMeas.Temprature", "SPMeas.Strobe_code", "SPMeas.HV_bias": Value Change {
        w342 = T19[] [enum."Meas.Grid update"] items=["idle", "HW.Conect", "HW.FreqC selftest", "HW.8164B selftest", "HW.Scope selftest", "HW.KC705 selftest", "HW.Laser test", "HW.Power source test", "SPD.connect", "SPD.set type", "SPD.write", "SPD.read", "SPD.tests", "Btf.DT&Insens", "Meas.Grid update", "Meas", "App.Handle Error", "App.Stop"] ("Array")
        n199 = event-data() -> ()  [unwired: 1 in, 3 out]
        n200 = call "SPD.Enqueue States.vi"("Error In"=w340, "SPD.states"=w342, "SPD.Stand Ctrl in"=w341) -> ("Error Out"=w339:errorcluster)  [unwired: 7 in, 1 out]
      }
      event "Meas": Value Change {
        w346 = T19[] [] items=["idle", "HW.Conect", "HW.FreqC selftest", "HW.8164B selftest", "HW.Scope selftest", "HW.KC705 selftest", "HW.Laser test", "HW.Power source test", "SPD.connect", "SPD.set type", "SPD.write", "SPD.read", "SPD.tests", "Btf.DT&Insens", "Meas.Grid update", "Meas", "App.Handle Error", "App.Stop"] ("f")
        w349 = T19[] [enum."Meas.Grid update", enum."Meas"] items=["idle", "HW.Conect", "HW.FreqC selftest", "HW.8164B selftest", "HW.Scope selftest", "HW.KC705 selftest", "HW.Laser test", "HW.Power source test", "SPD.connect", "SPD.set type", "SPD.write", "SPD.read", "SPD.tests", "Btf.DT&Insens", "Meas.Grid update", "Meas", "App.Handle Error", "App.Stop"] ("Array")
        n201 = event-data() -> ("NewVal"=w347:bool)  [unwired: 1 in]
        n202 = Select(t=w349, s=w347, f=w346) -> (s? t:f=w348:T19[])
        n203 = call "SPD.Enqueue States.vi"("Error In"=w350, "SPD.states"=w348, "SPD.Stand Ctrl in"=w351) -> ("Error Out"=w343:errorcluster)  [unwired: 7 in, 1 out]
        n204 = control-ref of="App.stop"() -> (w344:refnum<vi>)
        n205 = call "Enable Control.vi"("enable"=FALSE, "Control"=w344) -> ()  [unwired: 10 in]
      }
      event User Event; "App.stop": Value Change {
        w356 = T19[] [enum."App.Stop"] items=["idle", "HW.Conect", "HW.FreqC selftest", "HW.8164B selftest", "HW.Scope selftest", "HW.KC705 selftest", "HW.Laser test", "HW.Power source test", "SPD.connect", "SPD.set type", "SPD.write", "SPD.read", "SPD.tests", "Btf.DT&Insens", "Meas.Grid update", "Meas", "App.Handle Error", "App.Stop"] ("Array")
        n206 = event-data() -> ()  [unwired: 1 in, 1 out]
        n207 = call "SPD.Enqueue States.vi"("Error In"=w354, "SPD.states"=w356, "SPD.Stand Ctrl in"=w355) -> ("Error Out"=w352:errorcluster)  [unwired: 7 in, 1 out]
      }
      event Panel Close? {
        n208 = event-data() -> ()  [unwired: 1 in, 4 out]
        n209 = control-ref of="App.stop"() -> (w364:refnum<vi>)
        n210 = property class="Bool"(reference=w364) -> ("DisabledEnum"=w363:T18)  [unwired: 1 in, 2 out]
        n211 = Not Equal?(x=w363, y=T18."Enabled") -> (x != y?=w361:bool)
        n212 = case shown="True" w361 {
          tunnel: w360 -> [w366 w371]
          tunnel: w359 -> [w369 _]
          tunnel: [w365 w371] -> w357
          frame False {
            n213 = Unbundle By Name(w369) -> ("Events.Stop"=w368:refnum<user-event>)
            n214 = Generate User Event(user event=w368, event data cluster=TRUE ("event data"), error in=w366) -> (error out=w365:errorcluster)  [unwired: 1 in, 1 out]
          }
          frame True {
            n215 = One Button Dialog(message="Перед выходом\nостановите все измерения") -> ()  [unwired: 1 in, 1 out]
          }
        }
        n216 = event-data("Discard?"=TRUE) -> ()  [unwired: 1 in, 1 out]
      }
    }
  }
  n217 = Merge Errors(w18, w39) -> (w19:errorcluster)
  n218 = Unbundle By Name(w32) -> ("SPD.Result"=→"SPD.Result":T21)
  n219 = call "Destroy Events.vi"("Error In"=w19, "SPD.Stand Ctrl in"=w32) -> ("Error Out"=w26:errorcluster, "SPD.Stand Ctrl out"=w27:T4)  [unwired: 8 in]
  n220 = call "SPD.Release Queues.vi"("Error In"=w26, "SPD.Stand Ctrl in"=w27) -> ("Error Out"=w24:errorcluster, "SPD.Stand Ctrl out"=w25:T4)  [unwired: 8 in]
  n221 = call "SPD.Close Config File.vi"("Error In"=w24, "SPD.Stand Ctrl in"=w25) -> ("Error Out"=w34:errorcluster)  [unwired: 8 in, 1 out]
  n222 = Unregister For Events(event registration refnum=w21, error in=w34) -> (error out=→"Error Out":errorcluster)
  "test tabs" <- SPD.Stand_Tabs."Equipment" ("test tabs")
  "Console" <- "" ("Console")
